vi "InsOtherRead_ver1.0.vi"(0 "VISA session":refnum<visa-resource-name>, 1 "error out":errorcluster) -> (2 "VISA session 2":refnum<visa-resource-name>, 3 "Numeric":dbl, 4 "error out 2":errorcluster)   [LabVIEW 2012]
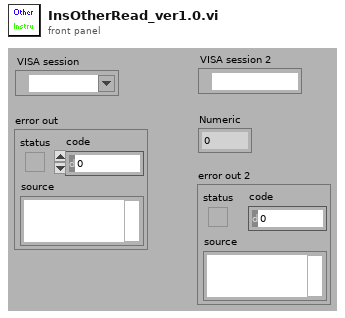
[diagram p1: front panel]
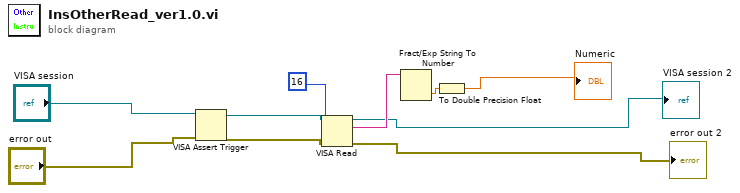
[diagram p0: block diagram]
diagram:
  n1 = VISA Assert Trigger(8:"error out", 11:"VISA session") -> (0:w3:errorcluster, 3:w4:refnum<visa-resource-name>)  [unwired: 1 in]
  n2 = VISA Read(VISA resource name=w4, byte count=u32 16, error in (no error)=w3) -> (VISA resource name out=→"VISA session 2":refnum<visa-resource-name>, read buffer=w10:string, error out=→"error out 2":errorcluster)  [unwired: 1 out]
  n3 = Fract/Exp String To Number(string=w10) -> (number=w9:dbl)  [unwired: 3 in, 1 out]
  n4 = To Double Precision Float(number=w9) -> (double precision float=→"Numeric":dbl)
